vi "Get Refs on Tabs (SubVI).vi"(8 "error in (no error)":errorcluster, 11 "Pages":refnum<vi>[](array[refnum])) -> (0 "error out":errorcluster, 2 "Refs":refnum<vi>[](array[refnum]), 3 "Labels":string[](array[string]))   [LabVIEW 2012]
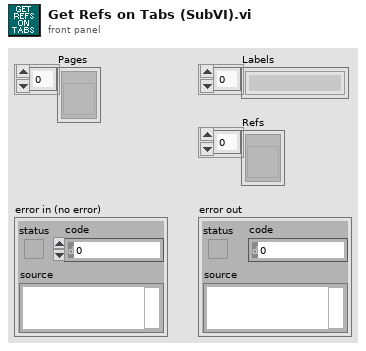
[diagram p1: front panel]
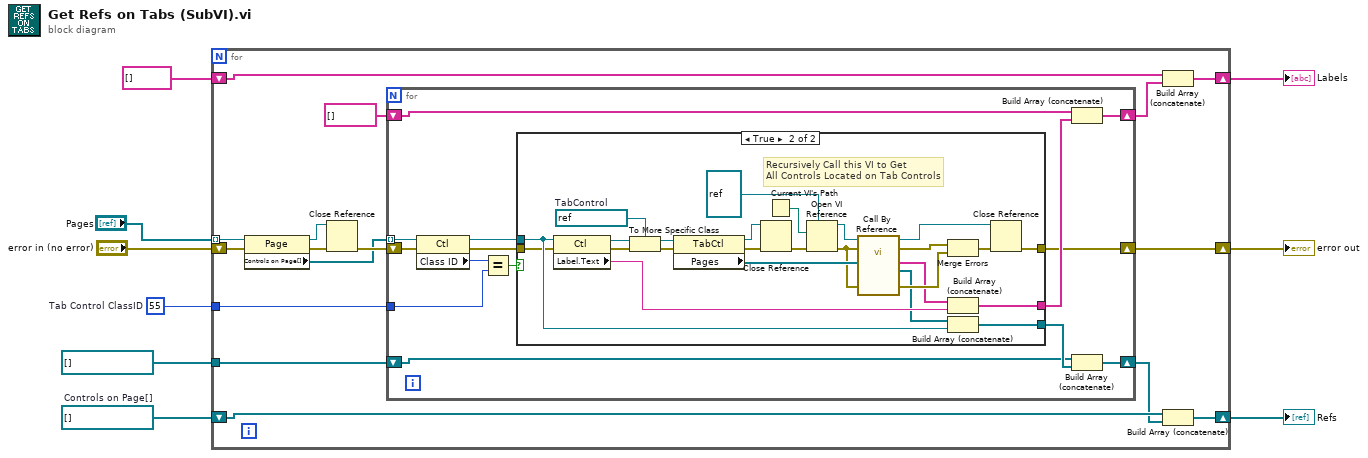
[diagram p0: block diagram]
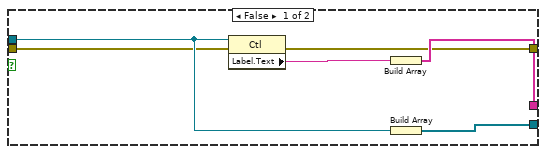
[diagram p2: hidden frame]
diagram:
  w3 = refnum<vi>[] []  # Controls on Page[]
  w8 = u32 55  # Tab Control ClassID
  n1 = for {
    tunnel: "Pages" -> [w25] mode=indexing
    shift-right: [w24] -> w4
    shift-left: string[] [] -> [w23]
    shift-right: [w22] -> w5
    shift-left: w3 -> [w21]
    shift-right: [w16] -> w7
    shift-left: "error in (no error)" -> [w17]
    tunnel: w8 -> [w15]
    tunnel: refnum<vi>[] [] -> [w10]
    n2 = property class="Page"(reference=w25, error in=w17) -> (reference out=w14:refnum<vi>, error out=w13:errorcluster, "Controls on Page[]"=w11:refnum<vi>[])
    n3 = Close Reference(reference=w14, error in (no error)=w13) -> (error out=w12:errorcluster)
    n4 = for {
      tunnel: w11 -> [w39] mode=indexing
      shift-right: [w31] -> w19
      shift-left: string[] [] -> [w33]
      shift-right: [w36] -> w20
      shift-left: w10 -> [w34]
      shift-right: [w27] -> w16
      shift-left: w12 -> [w29]
      tunnel: w15 -> [w26]
      n5 = property class="Ctl"(reference=w39, error in=w29) -> (reference out=w30:refnum<vi>, error out=w28:errorcluster, "Class ID"=w38:u32)
      n6 = Equal?(x=w38, y=w26) -> (x = y?=w37:bool)
      n7 = case shown="True" w37 {
        tunnel: w30 -> [w44 w65]
        tunnel: [w45 w67] -> w35
        tunnel: [w42 w63] -> w32
        tunnel: w28 -> [w41 w62]
        tunnel: [w40 w52] -> w27
        frame False {
          n8 = property class="Ctl"(reference=w44, error in=w41) -> (error out=w40:errorcluster, "Label.Text"=w43:string)  [unwired: 1 out]
          n9 = Build Array(w43) -> (w42:string[])
          n10 = Build Array(w44) -> (w45:refnum<vi>[])
        }
        frame True {
          w68 = refnum<vi> refnum  # TabControl
          # "Recursively Call this VI to Get \nAll Controls Located on Tab Controls"
          n11 = property class="Ctl"(reference=w65, error in=w62) -> (error out=w53:errorcluster, "Label.Text"=w64:string)  [unwired: 1 out]
          n12 = To More Specific Class(target class=w68, reference=w65, error in=w53) -> (specific class reference=w66:refnum<vi>, error out=w54:errorcluster)
          n13 = property class="TabCtl"(reference=w66, error in=w54) -> (reference out=w48:refnum<vi>, error out=w47:errorcluster, "Pages"=w57:refnum<vi>[])
          n14 = Close Reference(reference=w48, error in (no error)=w47) -> (error out=w46:errorcluster)
          n15 = Current VI's Path() -> (path=w59:path)
          n16 = Open VI Reference(type specifier VI Refnum (for type only)=refnum<vi> refnum, vi path=w59, error in (no error)=w46) -> (vi reference=w61:refnum<vi>, error out=w51:errorcluster)  [unwired: 3 in]
          n17 = call-by-ref "?"(reference=w61, error in=w51, "error in"=w51, "Pages"=w57) -> (reference out=w60:refnum<vi>, error out=w50:errorcluster, 0:"error out"=w69:errorcluster, "Cntrl Ref"=w55:refnum<vi>[], "Cntrl Labels"=w56:string[])  [unwired: 7 in]
          n18 = Merge Errors(w50, w69) -> (w49:errorcluster)
          n19 = Build Array (concatenate)(w56, w64) -> (w63:string[])
          n20 = Build Array (concatenate)(w55, w65) -> (w67:refnum<vi>[])
          n21 = Close Reference(reference=w60, error in (no error)=w49) -> (error out=w52:errorcluster)
        }
      }
      n22 = Build Array (concatenate)(w33, w32) -> (w31:string[])
      n23 = Build Array (concatenate)(w34, w35) -> (w36:refnum<vi>[])
    }
    n24 = Build Array (concatenate)(w23, w19) -> (w24:string[])
    n25 = Build Array (concatenate)(w21, w20) -> (w22:refnum<vi>[])
  }
  "Labels" <- w4
  "Refs" <- w5
  "error out" <- w7
